vi "Initialize_K6221.vi"   [LabVIEW 2018]
uses:
  Global Variables/global.vi
  Global Variables/Data_Display_global.vi
  Monitors/Utility/Monitor Communication/sub-vis/K6221_Open_Queue.vi
types:
  T1 = typedef "K6221_Cluster.ctl" = cluster{"Plot Window":dbl[][], "A":dbl, "A (RMS)":dbl, "Hz":dbl, "I (A)":dbl, "f (Hz)":dbl, "Update":bool, "Offset":dbl, "Offset (A)":dbl, "Compliance":bool, "Output":bool, "Output Status":bool}
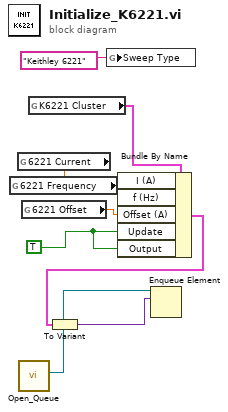
[diagram p0: block diagram]
diagram:
  w4 = TRUE
  n1 = global read "global.vi" "6221 Frequency"() -> (w2:dbl)
  n2 = global read "global.vi" "6221 Current"() -> (w3:dbl)
  n3 = call-poly "Open_Queue.vi"() -> ("queue out"=w7:refnum<queue>)  [unwired: 10 in, 1 out]
  n4 = global read "global.vi" "6221 Offset"() -> (w1:dbl)
  n5 = global read "Data_Display_global.vi" "K6221 Cluster"() -> (w8:T1)
  n6 = global write "global.vi" "Sweep Type"("Keithley 6221") -> ()
  n7 = Bundle By Name(cluster=w8, "I (A)"=w3, "f (Hz)"=w2, "Offset (A)"=w1, "Update"=w4, "Output"=w4) -> (w6:T1)
  n8 = To Variant(anything=w6) -> (Variant=w5:variant)
  n9 = Enqueue Element(queue=w7, element=w5) -> ()  [unwired: 2 in, 3 out]
